vi "Laser Power Ctrl Enable Setup Controls.vi"(2 "Enabled?":bool, 7 "Generic Class Ref":refnum<vi>, 13 "VI Path":path) -> ()   [LabVIEW 2016]
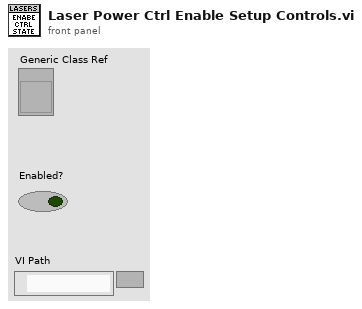
[diagram p1: front panel]
types:
  T1 = enum8{"Enabled", "Disabled", "Disabled and Grayed Out"}
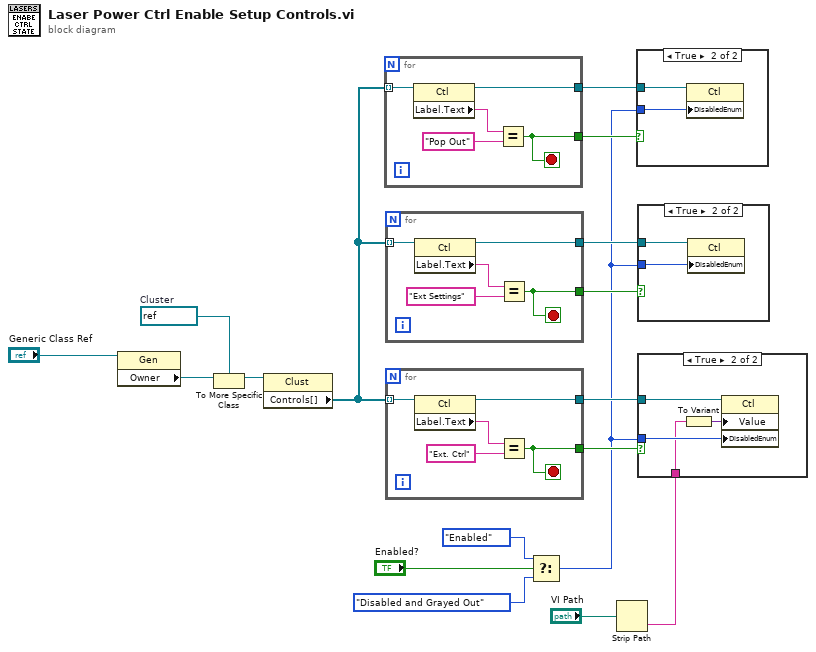
[diagram p0: block diagram]
diagram:
  w10 = refnum<vi> refnum  # Cluster
  n1 = property class="Gen"(reference="Generic Class Ref") -> ("Owner"=w9:refnum<vi>)  [unwired: 1 in, 2 out]
  n2 = To More Specific Class(target class=w10, reference=w9) -> (specific class reference=w7:refnum<vi>)  [unwired: 1 in, 1 out]
  n3 = property class="Clust"(reference=w7) -> ("Controls[]"=w2:refnum<vi>[])  [unwired: 1 in, 2 out]
  n4 = for {
    tunnel: w2 -> [w22] mode=indexing
    tunnel: [w19] -> w3
    tunnel: [w18] -> w4
    stop <- w19 stop-if-true
    n5 = property class="Ctl"(reference=w22) -> (reference out=w18:refnum<vi>, "Label.Text"=w21:string)  [unwired: 1 in, 1 out]
    n6 = Equal?(x=w21, y="Pop Out") -> (x = y?=w19:bool)
  }
  n7 = for {
    tunnel: w2 -> [w27] mode=indexing
    tunnel: [w24] -> w17
    tunnel: [w23] -> w16
    stop <- w24 stop-if-true
    n8 = property class="Ctl"(reference=w27) -> (reference out=w23:refnum<vi>, "Label.Text"=w26:string)  [unwired: 1 in, 1 out]
    n9 = Equal?(x=w26, y="Ext Settings") -> (x = y?=w24:bool)
  }
  n10 = for {
    tunnel: w2 -> [w32] mode=indexing
    tunnel: [w29] -> w11
    tunnel: [w28] -> w12
    stop <- w29 stop-if-true
    n11 = property class="Ctl"(reference=w32) -> (reference out=w28:refnum<vi>, "Label.Text"=w31:string)  [unwired: 1 in, 1 out]
    n12 = Equal?(x=w31, y="Ext. Ctrl") -> (x = y?=w29:bool)
  }
  n13 = Select(t=T1."Enabled" ("Disabled"), s="Enabled?", f=T1."Disabled and Grayed Out" ("Disabled")) -> (s? t:f=w1:T1)
  n14 = Strip Path(path="VI Path") -> (name=w5:string)  [unwired: 1 out]
  n15 = case shown="True" w3 {
    tunnel: w4 -> [_ w34]
    tunnel: w1 -> [_ w33]
    frame False {
    }
    frame True {
      n16 = property class="Ctl"(reference=w34, "DisabledEnum"=w33) -> ()  [unwired: 1 in, 2 out]
    }
  }
  n17 = case shown="True" w17 {
    tunnel: w16 -> [_ w36]
    tunnel: w1 -> [_ w35]
    frame False {
    }
    frame True {
      n18 = property class="Ctl"(reference=w36, "DisabledEnum"=w35) -> ()  [unwired: 1 in, 2 out]
    }
  }
  n19 = case shown="True" w11 {
    tunnel: w12 -> [_ w40]
    tunnel: w1 -> [_ w38]
    tunnel: w5 -> [_ w37]
    frame False {
    }
    frame True {
      n20 = To Variant(anything=w37) -> (Variant=w39:variant)
      n21 = property class="Ctl"(reference=w40, "Value"=w39, "DisabledEnum"=w38) -> ()  [unwired: 1 in, 2 out]
    }
  }
